vi "Diagnostics - Workspace Object.vi"() -> ()   [LabVIEW 2015, in "Diagnostics Workspace Object.lvlib"]
doc: "Sample numeric display item."
uses:
  Diagnostics Workspace Object.lvlib
  <vilib>/NI Veristand/Display Template Support/Display Template Support.llb/cluster_Screen Item Settings.ctl
  <vilib>/NI Veristand/Display Template Support/Display Template Support.llb/cluster_Graph Scale Settings.ctl
  <vilib>/NI Veristand/Display Template Support/Display Template Support.llb/cluster_Graph Plot Settings.ctl
  NationalInstruments.VeriStand.SystemStorage
  Shared/Types/Channel Commands Enum.ctl
  <vilib>/NI Veristand/Display Template Support/Display Template Support.llb/enum_Display Template Handler Minimal To Widget Msg.ctl
  <vilib>/NI Veristand/Display Template Support/Display Template Support.llb/enum_Display Template Handler Minimal To Workspace.ctl
  Shared/Types/Workspace Object State Variables.ctl
  Shared/Types/UI.Refs.ctl
  Shared/Types/CD Saved State.ctl
  <vilib>/NI Veristand/Execution/Workspace/WorkspaceAPI.ctl
  <vilib>/NI Veristand/Execution/Workspace/SystemStateRegEventRef.ctl
  <vilib>/NI Veristand/Execution/Workspace/Target State Info.ctl
  <vilib>/NI Veristand/Execution/Workspace/Target State.ctl
  <vilib>/NI Veristand/Execution/Workspace/SystemStateEventRef.ctl
  Shared/Types/Diagnostic Protocols.ctl
  <vilib>/NI Veristand/Display Template Support/Display Template Support.llb/sub_Display Template Handler Custom.vi
  <vilib>/NI Veristand/Execution/Workspace/NI VeriStand - Set Multiple Channel Values.vi
  <vilib>/NI Veristand/Execution/Workspace/NI VeriStand - Get Multiple Channel Values.vi
  <vilib>/NI Veristand/Execution/Workspace/NI_VS Workspace ExecutionAPI.lvlib
  Shared/Diagnostics Addon Shared.lvlib
  Automation API/Diagnostics Host Automation API.lvlib
  NationalInstruments.VeriStand.ClientAPI
panel:
  in  "Tab Control":enum32{"Cmd", "Raw"}(tab)
  in  "Send":bool
  out "Data Length":i64
  out "VeriStand Error":i64 format="%.0x"
  out "Error Byte":i64 format="%.0x"
  out "Success?":bool
  in  "MetaData1":i64 format="%.0x"
  in  "MetaData2":i64 format="%.0x"
  in  "MetaData3":i64 format="%.0x"
  in  "MetaData4":i64 format="%.0x"
  in  "Cmd":T1
  in  "Clear":bool
  out "VeriStand Error":errorcluster
  out "Error Byte":u8 format="%.0x"
  in  "Response Required?":bool
  in  "Send Raw":bool
  out "Resp":u8[](array[numeric]) format="%.0x"
  in  "Cmd":u8[](array[numeric]) format="%.0x"
  in  "NIVS.System Definition Root":refnum<k24>
  in  "NIVS.Gateway IP Address":string
  out "Control Name":string
  in  "Item.Data":T2
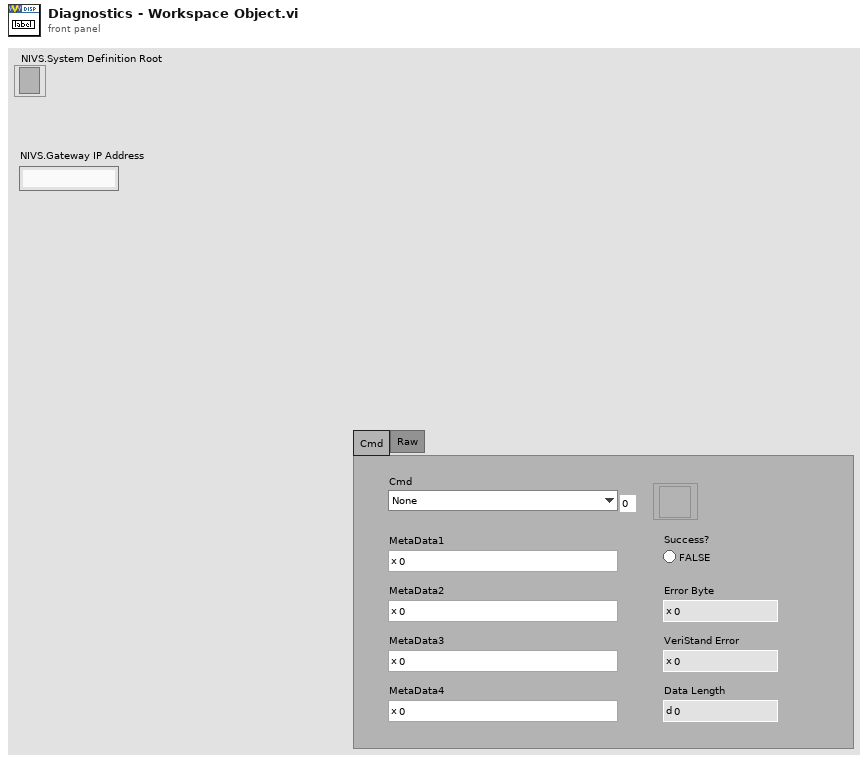
[diagram p1: front panel]
types:
  T1 = typedef "Diagnostics Addon Shared.lvlib/Channel Commands Enum.ctl" = enum8{"None", "EnableDiagnosticSession", "DisableDiagnosticSession", "ReadDataIdentifiers", "ReadDataIdentifier", "WriteDataIndentifier", "ReadPIDsOnDemand", "ReadPIDOnDemand", "WriteCPID", "WriteMemory", "ReadMemory", "ReadDTCs", "ClearDTCs", "ControlDTC", "ForceTesterPresent", "DisableNormalCommunication", "ReturnToNormalMode", "InputOutputControl", "StartRoutine", "RequestRoutineStatus", "StopRoutine", "ECUReset", "UnlockECU", "ClearSuccessBit", "ConfigureandStartPIDs", "StopPIDs", "StartDTCs", "EnableChangeDTCCount", "DisableChangeDTCCount", "ReadFailureRecordParameters", "PassThru Channel Based"}
  T2 = typedef "cluster_Screen Item Settings.ctl" = cluster{"Template VI":string, "Position X":i32, "Position Y":i32, "Custom":string, "Show Title Bar":bool, "ID":i32, "Always On Top":bool, "Allow Resize":bool, "Allow Minimize":bool, "Allow Close":bool, "Size to Screen":bool, "Screen.ID":i32, "State":enum16{"Normal", "New"}, "Title":string, "Window Bounds":cluster{"[0]":i16, "[1]":i16, "[2]":i16, "[3]":i16}, "Channel Ref":u64, "Unit":string, "Default Units?":bool, "Flash Limit?":bool, "Color 1":u32, "Color 2":u32, "Color 3":u32, "Color 4":u32, "Bck Color":u32, "Fore Color":u32, "Limit 1":dbl, "Limit 2":dbl, "Limit 3":dbl, "Limit 4":dbl, "Limit Mode 1":i32, "Limit Mode 2":i32, "Limit Mode 3":i32, "Limit Mode 4":i32, "Scale Precision":i32, "Scale Min":dbl, "Scale Max":dbl, "Format":i32, "Precision":i32, "Background Type":i32, "IDs":i32[], "Units":string[], "Labels":string[], "Scale Factor":dbl, "Scale Offset":dbl, "YScale Index":u32[], "XScale":T3, "YScales":T3[], "Plots":T4[], "Update Period":dbl, "History Length":dbl, "My.Ref":refnum<vi>, "Is Control?":bool, "Channel Paths":string[], "Custom Data":variant}
  T3 = typedef "cluster_Graph Scale Settings.ctl" = cluster{"Format":u8, "Precision":u8, "Fit":u8, "Label":string, "Use Default Label":bool, "Label Visible":bool, "Min":dbl, "Max":dbl}
  T4 = typedef "cluster_Graph Plot Settings.ctl" = cluster{"Bar Style":u8, "Fill To":i16, "Fill/PtColor":u32, "Line Style":u8, "Line Width":u8, "Color":u32, "Interp":u8, "Point Style":u8}
  T5 = typedef "Diagnostics Addon Shared.lvlib/Workspace Object State Variables.ctl" = cluster{"UI.Refs":T6, "Data.PreviousValues":dbl[], "Data.Read":string[], "CachedData.UserEvent":refnum<user-event>, "CachedData":T7, "Workspace.Connected?":bool, "NIVS.SysDef":refnum<k24>, "NIVS.WorkspaceManager":T8, "NIVS.UserEventRefs":cluster{"Event Registration Refnum":refnum<event-registration>, "SystemChangeEventRef":T9, "NIVS.Workspace Event":refnum<event-registration>}, "NIVS.SystemStateRefs":T10, "NIVS.LaunchRef":refnum<user-event>, "Data.PendingChange?":bool, "Data.Write":string[], "Diagnostic Protocol":T11, "Channels.Found":bool}
  T6 = typedef "Diagnostics Addon Shared.lvlib/UI.Refs.ctl" = cluster{"Cmd":refnum<vi>, "MetaData1":refnum<vi>, "MetaData2":refnum<vi>, "MetaData3":refnum<vi>, "MetaData4":refnum<vi>, "Success?":refnum<vi>, "ErrorByte":refnum<vi>, "VeriStandError":refnum<vi>, "DataLength":refnum<vi>}
  T7 = typedef "Diagnostics Addon Shared.lvlib/CD Saved State.ctl" = cluster{"CD Path":string, "CD IP":string}
  T8 = typedef "NI_VS Workspace ExecutionAPI.lvlib/WorkspaceAPI.ctl" = refnum<k24>
  T9 = typedef "NI_VS Workspace ExecutionAPI.lvlib/SystemStateRegEventRef.ctl" = refnum<event-registration>
  T10 = typedef "NI_VS Workspace ExecutionAPI.lvlib/SystemStateEventRef.ctl" = cluster{"CustDatRef":refnum<user-event>, "EvtRef":refnum<k27>, "Target State User Event":refnum<user-event>}
  T11 = typedef "Diagnostics Addon Shared.lvlib/Diagnostic Protocols.ctl" = enum16{"GMLAN", "KWP-2000", "UDS"}
  T12 = typedef "enum_Display Template Handler Minimal To Workspace.ctl" = cluster{"Operation":enum16{"SetCustomData", "DeleteItem"}, "Data":variant}
  T13 = typedef "enum_Display Template Handler Minimal To Widget Msg.ctl" = enum16{"Stop", "LaunchConfigDialog"}
  T14 = cluster{"Event Registration Refnum":refnum<event-registration>, "SystemChangeEventRef":T9, "NIVS.Workspace Event":refnum<event-registration>}
  T15 = typedef "NI_VS Workspace ExecutionAPI.lvlib/SystemState.ctl" = u8
  T16 = typedef "stm_TCP Connection Info.ctl" = cluster{"connection ID":refnum<k5>, "Meta data":T17[]}
  T17 = typedef "stm_MetaDataElement.ctl" = string
  T18 = cluster{"resp":u8[], "error code":u8, "error out":errorcluster}
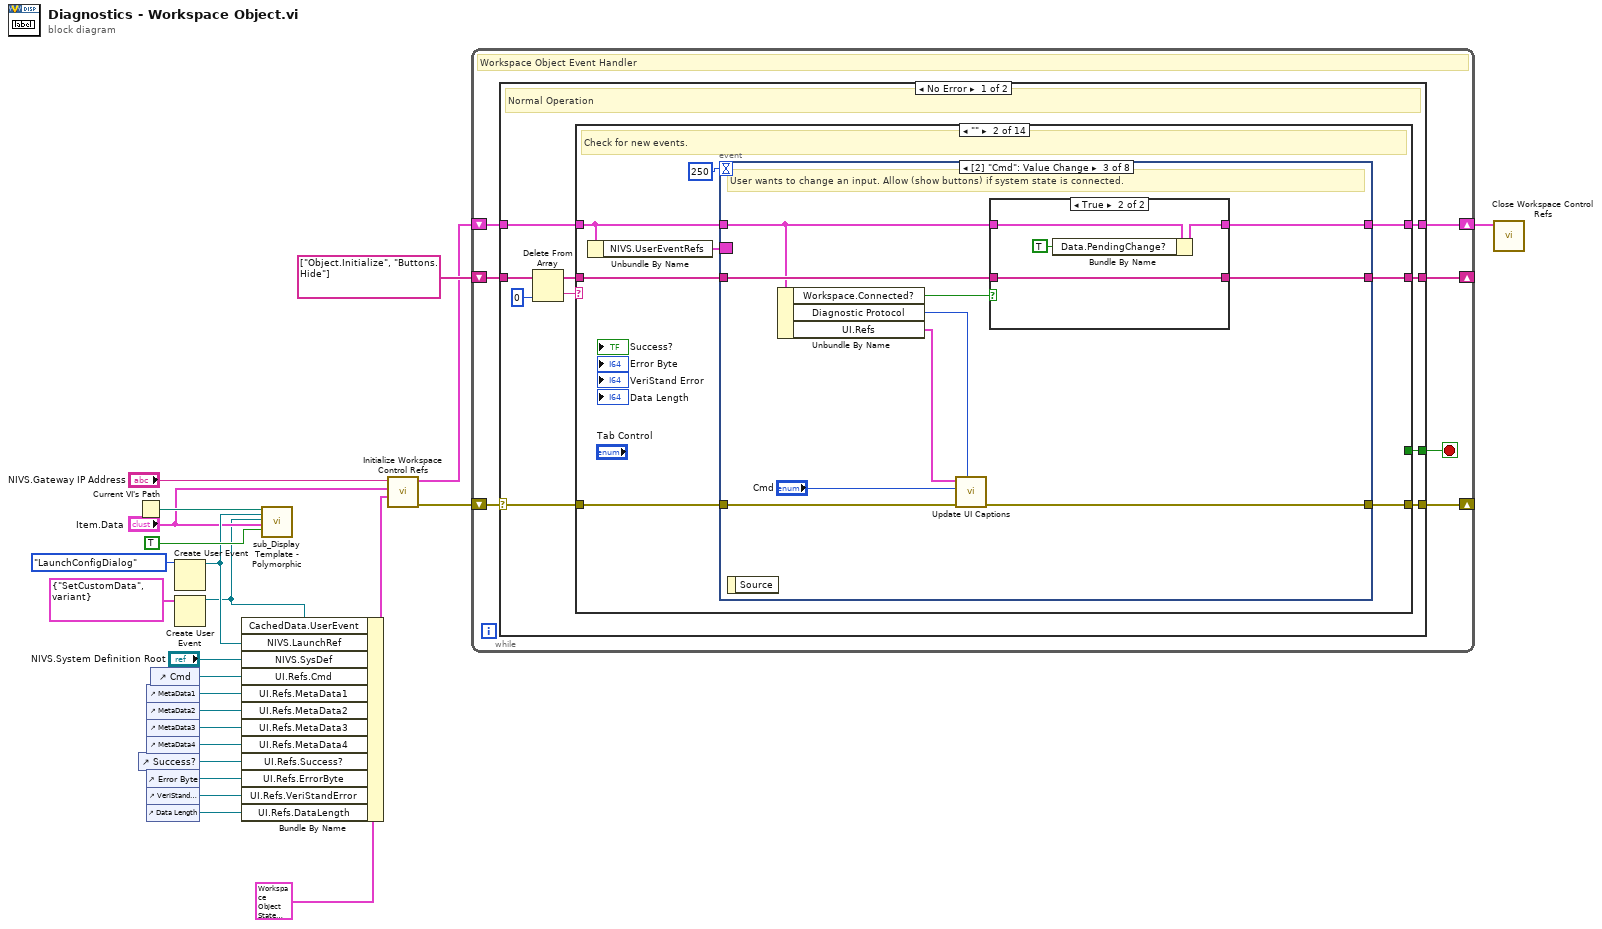
[diagram p0: block diagram]
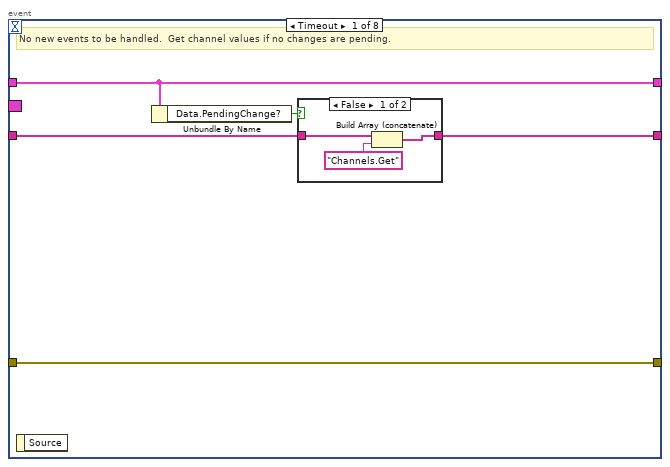
[diagram p3: hidden frame]
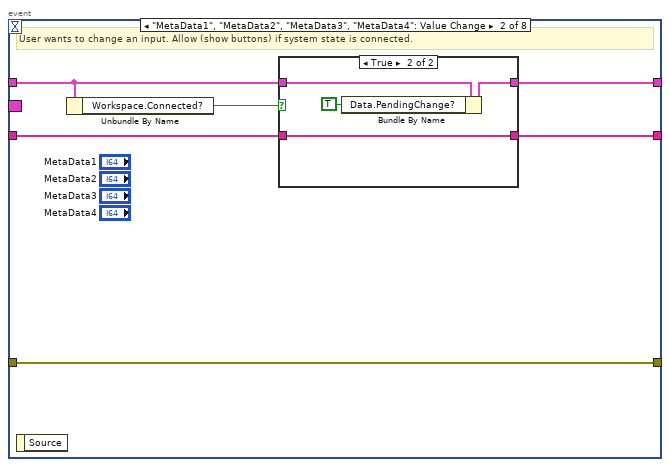
[diagram p5: hidden frame]
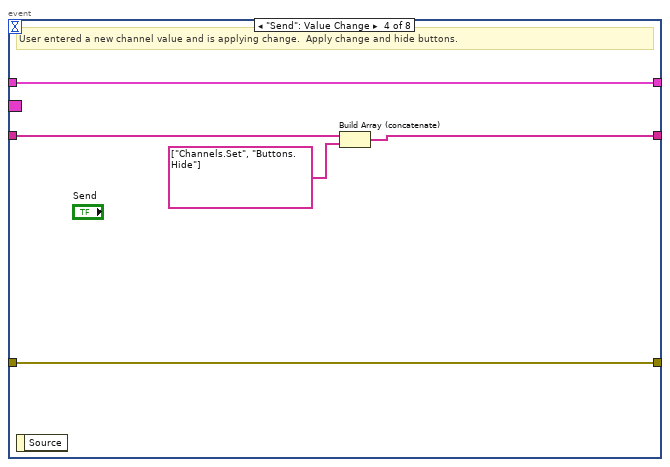
[diagram p8: hidden frame]
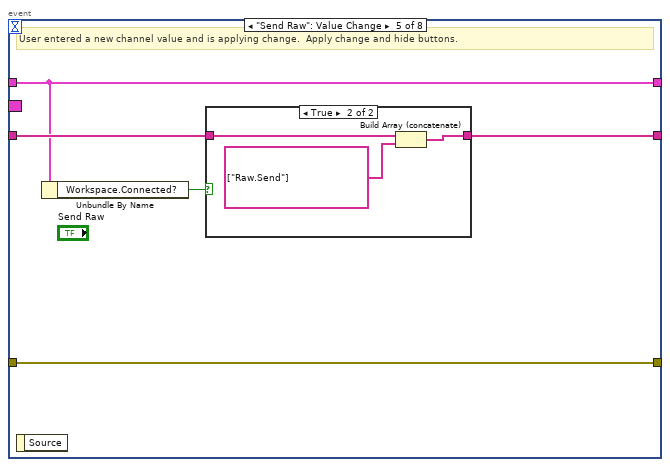
[diagram p9: hidden frame]
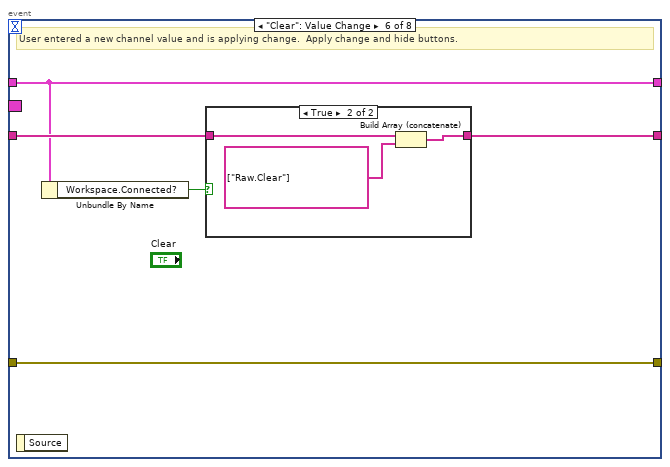
[diagram p11: hidden frame]
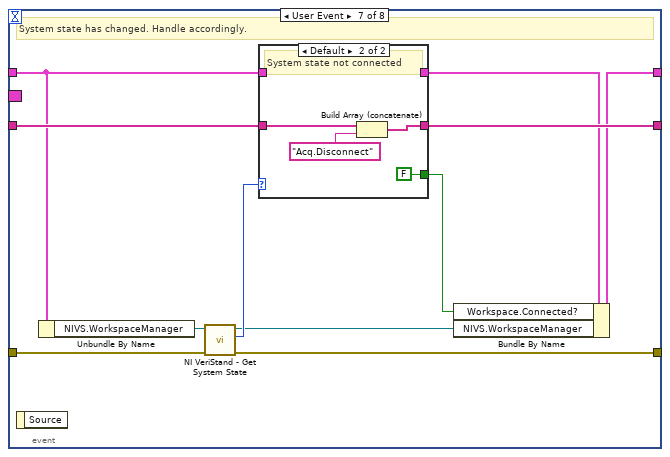
[diagram p13: hidden frame]
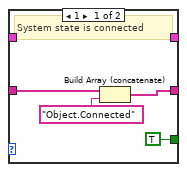
[diagram p14: hidden frame]
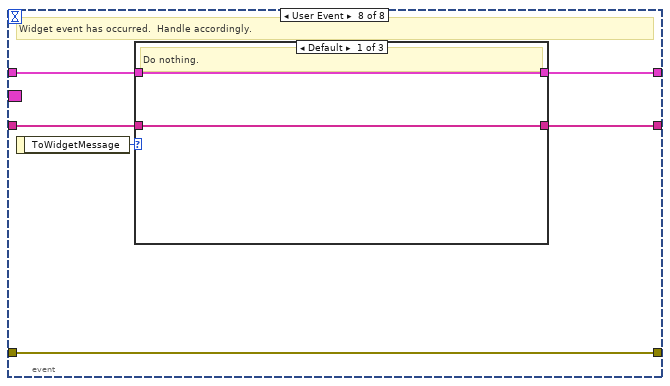
[diagram p15: hidden frame]
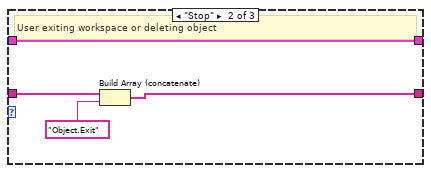
[diagram p16: hidden frame]
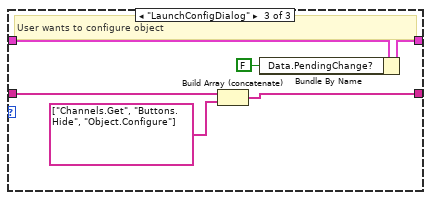
[diagram p17: hidden frame]
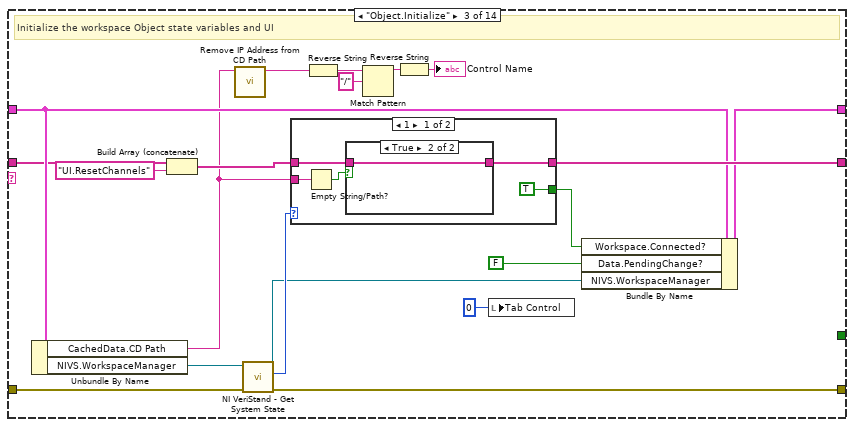
[diagram p18: hidden frame]
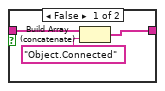
[diagram p19: hidden frame]
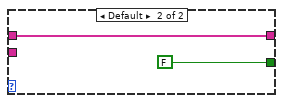
[diagram p20: hidden frame]
diagram:
  n1 = Current VI's Path() -> (path=w22:path)
  n2 = control-ref of="Success?"() -> (w2:refnum<vi>)
  n3 = control-ref of="MetaData1"() -> (w9:refnum<vi>)
  n4 = control-ref of="MetaData2"() -> (w8:refnum<vi>)
  n5 = control-ref of="MetaData3"() -> (w7:refnum<vi>)
  n6 = control-ref of="MetaData4"() -> (w6:refnum<vi>)
  n7 = control-ref of="Error Byte"() -> (w5:refnum<vi>)
  n8 = control-ref of="VeriStand Error"() -> (w4:refnum<vi>)
  n9 = control-ref of="Data Length"() -> (w3:refnum<vi>)
  n10 = control-ref of="Cmd"() -> (w1:refnum<vi>)
  n11 = Create User Event(user event datatype=enum_Display_Template_Handler_Minimal_To_Widget_Msg."LaunchConfigDialog" ("ToWidgetMessage")) -> (user event=w15:refnum<user-event>)  [unwired: 1 in, 1 out]
  n12 = Create User Event(user event datatype=T12 {"Operation"=enum."SetCustomData", "Data"=variant} ("Data")) -> (user event=w11:refnum<user-event>)  [unwired: 1 in, 1 out]
  n13 = Bundle By Name(cluster=T5 {"UI.Refs"={"Cmd"=refnum, "MetaData1"=refnum, "MetaData2"=refnum, "MetaData3"=refnum, "MetaData4"=refnum, "Success?"=refnum, "ErrorByte"=refnum, "VeriStandError"=refnum, "DataLength"=refnum}, "Data.PreviousValues"=[], "Data.Read"=[], "CachedData.UserEvent"=refnum, "CachedData"={"CD Path"="", "CD IP"=""}, "Workspace.Connected?"=FALSE, "NIVS.SysDef"=refnum, "NIVS.WorkspaceManager"=refnum, "NIVS.UserEventRefs"={"Event Registration Refnum"=refnum, "SystemChangeEventRef"=refnum, "NIVS.Workspace Event"=refnum}, "NIVS.SystemStateRefs"={"CustDatRef"=refnum, "EvtRef"=refnum, "Target State User Event"=refnum}, "NIVS.LaunchRef"=refnum, "Data.PendingChange?"=FALSE, "Data.Write"=[], "Diagnostic Protocol"=enum."GMLAN", "Channels.Found"=FALSE}, "CachedData.UserEvent"=w11, "NIVS.LaunchRef"=w15, "NIVS.SysDef"="NIVS.System Definition Root", "UI.Refs.Cmd"=w1, "UI.Refs.MetaData1"=w9, "UI.Refs.MetaData2"=w8, "UI.Refs.MetaData3"=w7, "UI.Refs.MetaData4"=w6, "UI.Refs.Success?"=w2, "UI.Refs.ErrorByte"=w5, "UI.Refs.VeriStandError"=w4, "UI.Refs.DataLength"=w3) -> (w13:T5)
  n14 = call-poly <vilib>:"sub_Display Template - Polymorphic.vi"("Parent.Path"=w22, "ToWidgetEvent"=w15, "ToWorkspace"=w11, "Item.Data"="Item.Data", "Resizable"=TRUE) -> ()  [unwired: 1 in, 14 out]
  n15 = call "Initialize Workspace Control Refs.vi"("State Variables in"=w13, "Item.Data"="Item.Data", "NIVS.Gateway IP Address"="NIVS.Gateway IP Address") -> ("error out"=w10:errorcluster, "State Variables out"=w17:T5)  [unwired: 7 in]
  n16 = while {
    shift-right: [w29] -> _
    shift-left: string[] ["Object.Initialize", "Buttons.Hide"] -> [w30]
    shift-right: [w27] -> w19
    shift-left: w17 -> [w26]
    shift-right: [w28] -> _
    shift-left: w10 -> [w25]
    stop <- w31 stop-if-true
    # "Workspace Object Event Handler"
    n17 = case shown="No Error" w25 {
      selector: w25 -> [w32 w314]
      tunnel: [w41 _] -> w31
      tunnel: w30 -> [w39 w321]
      tunnel: [w36 w321] -> w29
      tunnel: [w35 w312] -> w28
      tunnel: [w34 w320] -> w27
      tunnel: w26 -> [w33 w320]
      frame No Error {
        # "Normal Operation"
        n18 = Delete From Array(array=w39, index=0) -> (deleted portion=w38:string, array with subset deleted=w37:string[])  [unwired: 1 in]
        n19 = case shown="\"\"" w38 {
          tunnel: [_ _ _ _ _ TRUE _ _ _ _ _ _ _ _] -> w41
          tunnel: [w44 w51 w169 w186 w213 w221 w228 w231 w234 w243 w276 w289 w307 w311] -> w36
          tunnel: w32 -> [w43 w49 w170 w192 w209 w218 w227 w229 w232 w241 w275 w288 w306 w310]
          tunnel: w37 -> [w44 w50 w156 w185 w213 w221 w228 w231 w234 w243 w276 w289 w307 w311]
          tunnel: w33 -> [w42 w45 w161 w190 w215 w219 w224 w230 w233 w235 w273 w287 w303 w309]
          tunnel: [w43 w48 w154 w192 w208 w218 w227 w229 w232 w240 w274 w288 w306 w310] -> w35
          tunnel: [w42 w47 w164 w189 w214 w219 w224 w230 w233 w239 w272 w287 w303 w309] -> w34
          frame Default {
            # "Do nothing."
          }
          frame "" {
            # "Check for new events."
            n20 = Unbundle By Name(w45) -> ("NIVS.UserEventRefs"=w46:T14)
            n21 = event shown="[2] \"Cmd\": Value Change" {
              selector: w46 -> [_ _ _ _ _ _ _ _]
              dyn-events: _ -> [_ _ _ _ _ _ _ _]
              timeout: 250 -> [_ _ _ _ _ _ _ _]
              tunnel: [w55 w65 w81 w90 w97 w106 w119 w138] -> w51
              tunnel: w50 -> [w56 w66 w82 w91 w98 w107 w120 w137]
              tunnel: w49 -> [w57 w62 w78 w94 w99 w108 w123 w136]
              tunnel: [w57 w62 w77 w94 w99 w108 w122 w136] -> w48
              tunnel: [w54 w67 w83 w93 w96 w105 w118 w134] -> w47
              tunnel: w45 -> [w54 w64 w80 w93 w96 w105 w115 w135]
              event Timeout {
                # "No new events to be handled.  Get channel values if no changes are pending."
                n22 = event-data() -> ()  [unwired: 2 out]
                n23 = Unbundle By Name(w54) -> ("Data.PendingChange?"=w53:bool)
                n24 = case shown="False" w53 {
                  tunnel: w56 -> [w59 w61]
                  tunnel: [w58 w61] -> w55
                  frame False {
                    n25 = Build Array (concatenate)(w59, "Channels.Get") -> (w58:string[])
                  }
                  frame True {
                  }
                }
              }
              event "MetaData1", "MetaData2", "MetaData3", "MetaData4": Value Change {
                # "User wants to change an input. Allow (show buttons) if system state is connected."
                n26 = event-data() -> ()  [unwired: 2 out]
                n27 = Unbundle By Name(w64) -> ("Workspace.Connected?"=w63:bool)
                n28 = case shown="True" w63 {
                  tunnel: w64 -> [w68 w72]
                  tunnel: [w68 w71] -> w67
                  tunnel: w66 -> [w69 w70]
                  tunnel: [w69 w70] -> w65
                  frame False {
                  }
                  frame True {
                    n29 = Bundle By Name(cluster=w72, "Data.PendingChange?"=TRUE ("Pending Change?")) -> (w71:T5)
                  }
                }
              }
              event Value Change {
                # "User wants to change an input. Allow (show buttons) if system state is connected."
                n30 = event-data() -> ()  [unwired: 2 out]
                n31 = Unbundle By Name(w80) -> ("Workspace.Connected?"=w79:bool, "Diagnostic Protocol"=w74:T11, "UI.Refs"=w76:T6)
                n32 = call "Update UI Captions.vi"("Diagnostic Protocol"=w74, "error in (no error)"=w78, "Cmd"="Cmd", "UI.Refs"=w76) -> ("error out"=w77:errorcluster)  [unwired: 7 in]
                n33 = case shown="True" w79 {
                  tunnel: w80 -> [w84 w88]
                  tunnel: [w84 w87] -> w83
                  tunnel: w82 -> [w85 w86]
                  tunnel: [w85 w86] -> w81
                  frame False {
                  }
                  frame True {
                    n34 = Bundle By Name(cluster=w88, "Data.PendingChange?"=TRUE ("Pending Change?")) -> (w87:T5)
                  }
                }
              }
              event "Send": Value Change {
                # "User entered a new channel value and is applying change.  Apply change and hide buttons."
                n35 = event-data() -> ()  [unwired: 2 out]
                n36 = Build Array (concatenate)(w91, string[] ["Channels.Set", "Buttons.Hide"]) -> (w90:string[])
              }
              event "Send Raw": Value Change {
                # "User entered a new channel value and is applying change.  Apply change and hide buttons."
                n37 = event-data() -> ()  [unwired: 2 out]
                n38 = Unbundle By Name(w96) -> ("Workspace.Connected?"=w95:bool)
                n39 = case shown="True" w95 {
                  tunnel: w98 -> [w100 w102]
                  tunnel: [w100 w101] -> w97
                  frame False {
                  }
                  frame True {
                    n40 = Build Array (concatenate)(w102, string[] ["Raw.Send"]) -> (w101:string[])
                  }
                }
              }
              event "Clear": Value Change {
                # "User entered a new channel value and is applying change.  Apply change and hide buttons."
                n41 = event-data() -> ()  [unwired: 2 out]
                n42 = Unbundle By Name(w105) -> ("Workspace.Connected?"=w104:bool)
                n43 = case shown="True" w104 {
                  tunnel: w107 -> [w109 w111]
                  tunnel: [w109 w110] -> w106
                  frame False {
                  }
                  frame True {
                    n44 = Build Array (concatenate)(w111, string[] ["Raw.Clear"]) -> (w110:string[])
                  }
                }
              }
              event User Event {
                # "System state has changed. Handle accordingly."
                n45 = event-data() -> ()  [unwired: 2 out]
                n46 = Unbundle By Name(w115) -> ("NIVS.WorkspaceManager"=w114:T8)
                n47 = call <vilib>:"NI VeriStand - Get System State.vi"("error in (no error)"=w123, "WorkspaceManager in"=w114) -> ("error out"=w122:errorcluster, "System State"=w121:T15, "WorkspaceManager  out"=w113:T8)  [unwired: 5 in, 2 out]
                n48 = case shown="Default" w121 {
                  tunnel: w120 -> [w128 w133]
                  tunnel: [w127 w132] -> w119
                  tunnel: [w125 w130] -> w117
                  tunnel: w115 -> [w125 w130]
                  tunnel: [TRUE FALSE] -> w116
                  frame 1 {
                    # "System state is connected"
                    n49 = Build Array (concatenate)(w128, "Object.Connected") -> (w127:string[])
                  }
                  frame Default {
                    # "System state not connected"
                    n50 = Build Array (concatenate)(w133, "Acq.Disconnect") -> (w132:string[])
                  }
                }
                n51 = Bundle By Name(cluster=w117, "Workspace.Connected?"=w116, "NIVS.WorkspaceManager"=w113) -> (w118:T5)
              }
              event User Event {
                # "Widget event has occurred.  Handle accordingly."
                n52 = event-data() -> ("ToWidgetMessage"=w139:T13)  [unwired: 1 out]
                n53 = case shown="Default" w139 {
                  tunnel: [w141 w144 w150] -> w138
                  tunnel: w137 -> [w141 w145 w151]
                  tunnel: w135 -> [w140 w142 w147]
                  tunnel: [w140 w142 w146] -> w134
                  frame Default {
                    # "Do nothing."
                  }
                  frame "Stop" {
                    # "User exiting workspace or deleting object"
                    n54 = Build Array (concatenate)(w145, "Object.Exit") -> (w144:string[])
                  }
                  frame "LaunchConfigDialog" {
                    # "User wants to configure object"
                    n55 = Build Array (concatenate)(w151, string[] ["Channels.Get", "Buttons.Hide", "Object.Configure"]) -> (w150:string[])
                    n56 = Bundle By Name(cluster=w147, "Data.PendingChange?"=FALSE ("Pending Change?")) -> (w146:T5)
                  }
                }
              }
            }
          }
          frame "Object.Initialize" {
            # "Initialize the workspace Object state variables and UI"
            n57 = Unbundle By Name(w161) -> ("CachedData.CD Path"=w152:string, "NIVS.WorkspaceManager"=w160:T8)
            n58 = Build Array (concatenate)(w156, "UI.ResetChannels") -> (w155:string[])
            n59 = call "Remove IP Address from CD Path.vi"("CD Path"=w152) -> ("Path"=w158:string)  [unwired: 9 in, 1 out]
            n60 = call <vilib>:"NI VeriStand - Get System State.vi"("error in (no error)"=w170, "WorkspaceManager in"=w160) -> ("error out"=w154:errorcluster, "System State"=w171:T15, "WorkspaceManager  out"=w159:T8)  [unwired: 5 in, 2 out]
            n61 = case shown="1" w171 {
              tunnel: w155 -> [w176 w181]
              tunnel: [w175 w181] -> w169
              tunnel: [TRUE FALSE] -> w163
              tunnel: w152 -> [w173 _]
              frame 1 {
                n62 = Empty String/Path?(string/path=w173) -> (empty?=w172:bool)
                n63 = case shown="True" w172 {
                  tunnel: w176 -> [w179 w180]
                  tunnel: [w178 w180] -> w175
                  frame False {
                    n64 = Build Array (concatenate)(w179, "Object.Connected") -> (w178:string[])
                  }
                  frame True {
                  }
                }
              }
              frame Default {
              }
            }
            n65 = Reverse String(1:w158) -> (0:w168:string)
            n66 = Match Pattern(string=w168, regular expression="/") -> (before substring=w165:string)  [unwired: 1 in, 3 out]
            n67 = Reverse String(1:w165) -> (0:→"Control Name":string)
            n68 = local write "Tab Control"(0) -> ()
            n69 = Bundle By Name(cluster=w161, "Workspace.Connected?"=w163, "Data.PendingChange?"=FALSE ("Pending Change?"), "NIVS.WorkspaceManager"=w159) -> (w164:T5)
          }
          frame "Object.Configure" {
            # "Allow the user to select a control object to display"
            n70 = Unbundle By Name(w190) -> ("NIVS.SysDef"=w184:refnum<k24>, "CachedData.CD Path"=w191:string)
            n71 = call "Select Controller.vi"("CD Path"=w191, "NIVS.System Definition Root"=w184) -> ("Cancelled?"=w188:bool, "IP Address"=w183:string, "Custom Device Path Out"=w187:string)  [unwired: 7 in]
            n72 = case shown="False" w188 {
              tunnel: w190 -> [w199 w200]
              tunnel: [w198 w200] -> w189
              tunnel: w187 -> [w197 _]
              tunnel: [w195 w201] -> w186
              tunnel: w185 -> [w196 w201]
              tunnel: w183 -> [w193 _]
              frame False {
                # "Queue up required states and cache new controller path"
                n73 = Bundle By Name(cluster=w199, "CachedData.CD Path"=w197, "CachedData.CD IP"=w193) -> (w198:T5)
                n74 = Build Array (concatenate)(w196, string[] ["Cache.Update", "Object.Initialize"]) -> (w195:string[])
              }
              frame True {
                # "User canceled"
              }
            }
          }
          frame "Object.Connected" {
            # "System state is Connected. Get path to required channels and start UDP acquisition if channels found."
            n75 = Unbundle By Name(w215) -> ("CachedData.CD Path"=w207:string, "NIVS.SysDef"=w205:refnum<k24>, "UI.Refs.Cmd"=w203:refnum<vi>)
            n76 = call "Remove IP Address from CD Path.vi"("CD Path"=w207) -> ("Path"=w206:string)  [unwired: 9 in, 1 out]
            n77 = call "CreateChannelLists.vi"("CD Path"=w207) -> ("Read Channels"=w212:string[], "Write Channels"=w211:string[])  [unwired: 9 in]
            n78 = call "Get Controller Variables Ranges.vi"("error in (no error)"=w209, "Path"=w206, "NIVS.SysDef Ref"=w205) -> ("error out"=w210:errorcluster, "Diagnostic Protocol"=w204:T11)  [unwired: 7 in]
            n79 = case shown="\"GMLAN\"" w204 {
              tunnel: [w216 w217] -> w202
              frame "GMLAN" {
                w216 = T1[] [enum."ECUReset", enum."WriteMemory", enum."ReadMemory", enum."InputOutputControl", enum."StartRoutine", enum."RequestRoutineStatus", enum."StopRoutine", enum."ControlDTC", enum."ReadDTCs", enum."WriteDataIndentifier"] items=["None", "EnableDiagnosticSession", "DisableDiagnosticSession", "ReadDataIdentifiers", "ReadDataIdentifier", "WriteDataIndentifier", "ReadPIDsOnDemand", "ReadPIDOnDemand", "WriteCPID", "WriteMemory", "ReadMemory", "ReadDTCs", "ClearDTCs", "ControlDTC", "ForceTesterPresent", "DisableNormalCommunication", "ReturnToNormalMode", "InputOutputControl", "StartRoutine", "RequestRoutineStatus", "StopRoutine", "ECUReset", "UnlockECU", "ClearSuccessBit", "ConfigureandStartPIDs", "StopPIDs", "StartDTCs", "EnableChangeDTCCount", "DisableChangeDTCCount", "ReadFailureRecordParameters", "PassThru Channel Based"] ("Disabled Items []")
              }
              frame Default {
                w217 = T1[] [enum."EnableChangeDTCCount", enum."DisableChangeDTCCount", enum."StartDTCs", enum."ReadFailureRecordParameters", enum."ConfigureandStartPIDs", enum."StopPIDs", enum."WriteCPID", enum."ReadPIDsOnDemand", enum."ReadPIDOnDemand"] items=["None", "EnableDiagnosticSession", "DisableDiagnosticSession", "ReadDataIdentifiers", "ReadDataIdentifier", "WriteDataIndentifier", "ReadPIDsOnDemand", "ReadPIDOnDemand", "WriteCPID", "WriteMemory", "ReadMemory", "ReadDTCs", "ClearDTCs", "ControlDTC", "ForceTesterPresent", "DisableNormalCommunication", "ReturnToNormalMode", "InputOutputControl", "StartRoutine", "RequestRoutineStatus", "StopRoutine", "ECUReset", "UnlockECU", "ClearSuccessBit", "ConfigureandStartPIDs", "StopPIDs", "StartDTCs", "EnableChangeDTCCount", "DisableChangeDTCCount", "ReadFailureRecordParameters", "PassThru Channel Based"] ("Disabled Items []")
              }
            }
            n80 = Bundle By Name(cluster=w215, "Data.Write"=w211, "Data.Read"=w212, "Diagnostic Protocol"=w204) -> (w214:T5)
            n81 = property class="Enum (strict)"(reference=w203, error in=w210, "Disabled Items []"=w202) -> (error out=w208:errorcluster)  [unwired: 1 out]
          }
          frame "Object.Exit" {
            # "Stop current loop.  Queue Stop Acq and Exit to UDP loop."
          }
          frame "Cache.Update" {
            # "Cache any data needing to be permenantly stored with the workspace object."
            n82 = Unbundle By Name(w224) -> ("CachedData.UserEvent"=w222:refnum<user-event>, "CachedData"=w223:T7)
            n83 = Bundle By Name(cluster=T12 {"Operation"=enum."SetCustomData", "Data"=variant} ("event data"), "Data"=w223) -> (w225:T12)
            n84 = Generate User Event(user event=w222, event data cluster=w225) -> ()  [unwired: 2 in, 2 out]
          }
          frame "Buttons.Hide" {
            # "Hide the apply and revert buttons from the user."
          }
          frame "Buttons.Show" {
            # "Show the apply and revert buttons to the user."
          }
          frame "Channels.Get" {
            # "Get the current slow speed channel values from VeriStand if no pending change, data paths are valid and system state is connected."
            n85 = Unbundle By Name(w235) -> ("Data.PendingChange?"=w236:bool, "Workspace.Connected?"=w242:bool, "NIVS.WorkspaceManager"=w238:T8, "Data.Read"=w237:string[])
            n86 = case shown="False" w236 {
              tunnel: w242 -> [w249 _]
              tunnel: w241 -> [w254 w264]
              tunnel: [w244 w264] -> w240
              tunnel: [w253 w265] -> w239
              tunnel: w238 -> [w252 _]
              tunnel: w237 -> [w250 _]
              tunnel: w235 -> [w247 w265]
              frame False {
                # "No pending data change.  Allow for a get."
                n87 = case shown="True" w249 {
                  tunnel: w254 -> [w257 w263]
                  tunnel: [w257 w262] -> w245
                  tunnel: w252 -> [w256 w261]
                  tunnel: [w256 w260] -> w251
                  tunnel: w250 -> [_ w259]
                  tunnel: [dbl[] [0.0, 0.0, 0.0] ("Values") w258] -> w248
                  frame False {
                    # "Do Nothing."
                  }
                  frame True {
                    # "Connected & paths valid"
                    n88 = call-poly <vilib>:"NI VeriStand - Get Channel Value.vi"("error in (no error)"=w263, "Channels"=w259, "WorkspaceManager in"=w261) -> ("error out"=w262:errorcluster, "Values"=w258:dbl[], "WorkspaceManager out"=w260:T8)  [unwired: 6 in]
                  }
                }
                n89 = Unbundle By Name(w247) -> ("UI.Refs"=w246:T6)
                n90 = call "Workspace Update UI Objects.vi"("error in (no error)"=w245, "Values"=w248, "UI.Refs"=w246) -> ("error out"=w244:errorcluster)  [unwired: 8 in]
                n91 = Bundle By Name(cluster=w247, "NIVS.WorkspaceManager"=w251, "Data.PreviousValues"=w248) -> (w253:T5)
              }
              frame True {
                # "A change is pending.  Don't get channels as this would overwrite the pending change."
              }
            }
          }
          frame "Channels.Set" {
            # "Set Channels if data paths are valid and system state is connected and there is a change in the data value."
            n92 = Unbundle By Name(w273) -> ("Workspace.Connected?"=w269:bool, "NIVS.WorkspaceManager"=w268:T8, "Data.Write"=w266:string[], "UI.Refs"=w267:T6)
            n93 = case shown="True" w269 {
              tunnel: w275 -> [w278 w280]
              tunnel: [w278 w286] -> w274
              tunnel: w268 -> [w277 w285]
              tunnel: [w277 w284] -> w270
              tunnel: w266 -> [_ w283]
              tunnel: w267 -> [_ w281]
              frame False {
                # "Do nothing"
              }
              frame True {
                # "Connected & paths valid"
                n94 = call "Workspace Pull UI Objects.vi"("error in (no error)"=w280, "UI.Refs"=w281) -> ("error out"=w279:errorcluster, "Values"=w282:dbl[])  [unwired: 8 in]
                n95 = call-poly <vilib>:"NI VeriStand - Set Channel Value.vi"("error in (no error)"=w279, "Values"=w282, "Channels"=w283, "WorkspaceManager in"=w285) -> ("error out"=w286:errorcluster, "WorkspaceManager out"=w284:T8)  [unwired: 6 in]
              }
            }
            n96 = Bundle By Name(cluster=w273, "Data.PendingChange?"=FALSE ("Pending Change?"), "NIVS.WorkspaceManager"=w270) -> (w272:T5)
          }
          frame "UI.ResetChannels" {
            # "Reset slow speed channel displayed values."
          }
          frame "Raw.Send" {
            # "Reset slow speed channel displayed values."
            n97 = Unbundle By Name(w303) -> ("CachedData.CD IP"=w291:string, "CachedData.CD Path"=w302:string)
            n98 = call "Remove IP Address from CD Path.vi"("CD Path"=w302) -> ("Name"=w290:string)  [unwired: 9 in, 1 out]
            n99 = Bundle By Name(cluster=cluster{"cmd":u8[], "require response?":bool} {"cmd"=[], "require response?"=TRUE} ("Cmd"), "cmd"="Cmd", "require response?"="Response Required?") -> (w300:cluster{"cmd":u8[], "require response?":bool})
            n100 = call "Connect.vi"("Addon Name"=w290, "Address"=w291) -> ("error out"=w297:errorcluster, "Connection Info Out"=w304:T16)  [unwired: 8 in]
            n101 = call "PassThru.vi"("error in (no error)"=w297, "Cmd"=w300, "Connection Info"=w304) -> ("error out"=w296:errorcluster, "Resp"=w295:T18, "Connection Info"=w305:T16)  [unwired: 6 in]
            n102 = Unbundle By Name(w295) -> ("resp"=→"Resp":u8[], "error code"=→"Error Byte":u8, "error out"=→"VeriStand Error":errorcluster)
            n103 = call "Disconnect.vi"("error in"=w296, "Connection Info"=w305) -> ()  [unwired: 9 in, 1 out]
          }
          frame "Raw.Clear" {
            n104 = local write "Cmd"(u8[] [] ("Cmd")) -> ()
          }
        }
      }
      frame Error {
        # "Handle Errors."
        n105 = Unbundle By Name(w314) -> ("code"=w318:i32)
        n106 = Equal?(x=-307654, y=w318) -> (x = y?=w316:bool)
        n107 = Select(t=errorcluster {"status"=FALSE, "code"=0, "source"=""}, s=w316, f=w314) -> (s? t:f=w313:errorcluster)
        n108 = call <vilib>:"Simple Error Handler.vi"("error in (no error)"=w313) -> ("error out"=w319:errorcluster)  [unwired: 4 in, 4 out]
        n109 = call <vilib>:"Clear Errors.vi"("error in (no error)"=w319) -> ("error out"=w312:errorcluster)  [unwired: 5 in, 1 out]
      }
    }
  }
  n110 = call "Close Workspace Control Refs.vi"("State Variables in"=w19) -> ()  [unwired: 11 in]
